vi "Teleop.vi"(10 "Match Info":T1={"Autonomous Elapsed Seconds"=0.0, "TeleOp Elapsed Seconds"=0.0, "Disabled Elapsed Seconds"=0.0, "Visited Autonomous"=FALSE, "Visited TeleOp"=FALSE, "Visited Disabled"=FALSE, "Autonomous Settings"={"Autonomous Style"=enum."Independent", "VI Refnum"=refnum}}, 11 "Call Context":T2) -> ()   [LabVIEW 2018]
doc: "This VI is called for each enabled TeleOp packet received from the DS. It is typically used to read from joysticks and other inputs and update I/O or setpoints for timed control loops. It should complete and return within 20 milliseconds or risk missing DS packets."
uses:
  <vilib>/Rock Robotics/WPI/DriverStation/WPI_DriverStationDerivedRobotMode.ctl
  <vilib>/Rock Robotics/WPI/DriverStation/WPI_DriverStationMatch Info.ctl
  <vilib>/Rock Robotics/WPI/Solenoid/WPI_SolenoidValue.ctl
  Support Code/Climb State Machine Enum.ctl
  Framework/Robot Global Data.vi
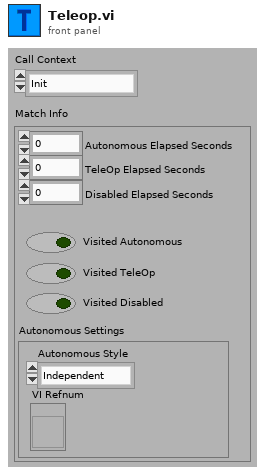
[diagram p1: front panel]
types:
  T1 = typedef "WPI_DriverStationMatch Info.ctl" = cluster{"Autonomous Elapsed Seconds":dbl, "TeleOp Elapsed Seconds":dbl, "Disabled Elapsed Seconds":dbl, "Visited Autonomous":bool, "Visited TeleOp":bool, "Visited Disabled":bool, "Autonomous Settings":cluster{"Autonomous Style":enum16{"Iterative", "Independent"}, "VI Refnum":refnum<vi>}}
  T2 = typedef "WPI_DriverStationDerivedRobotMode.ctl" = enum16{"Init", "Execute", "Stop"}
  T3 = typedef "WPI_SolenoidValue.ctl" = enum16{"Off", "On", "Forward", "Reverse"}
  T4 = typedef "Command Status Info.ctl" = cluster{"Name":string, "Status":T5, "notifier out":T6}
  T5 = typedef "Completion Status.ctl" = enum16{"Successful", "Aborted", "Incomplete"}
  T6 = typedef "Completion Notifier.ctl" = refnum<notifier>
  T7 = typedef "Climb State Machine Enum.ctl" = enum16{"Raise the front of the Robot", "Drive the front forward", "Lift the front pistons", "Lift the back of the Robot", "Drive the back of the robot forward", "Lift the back pistons", "Drive Forward", "Exit"}
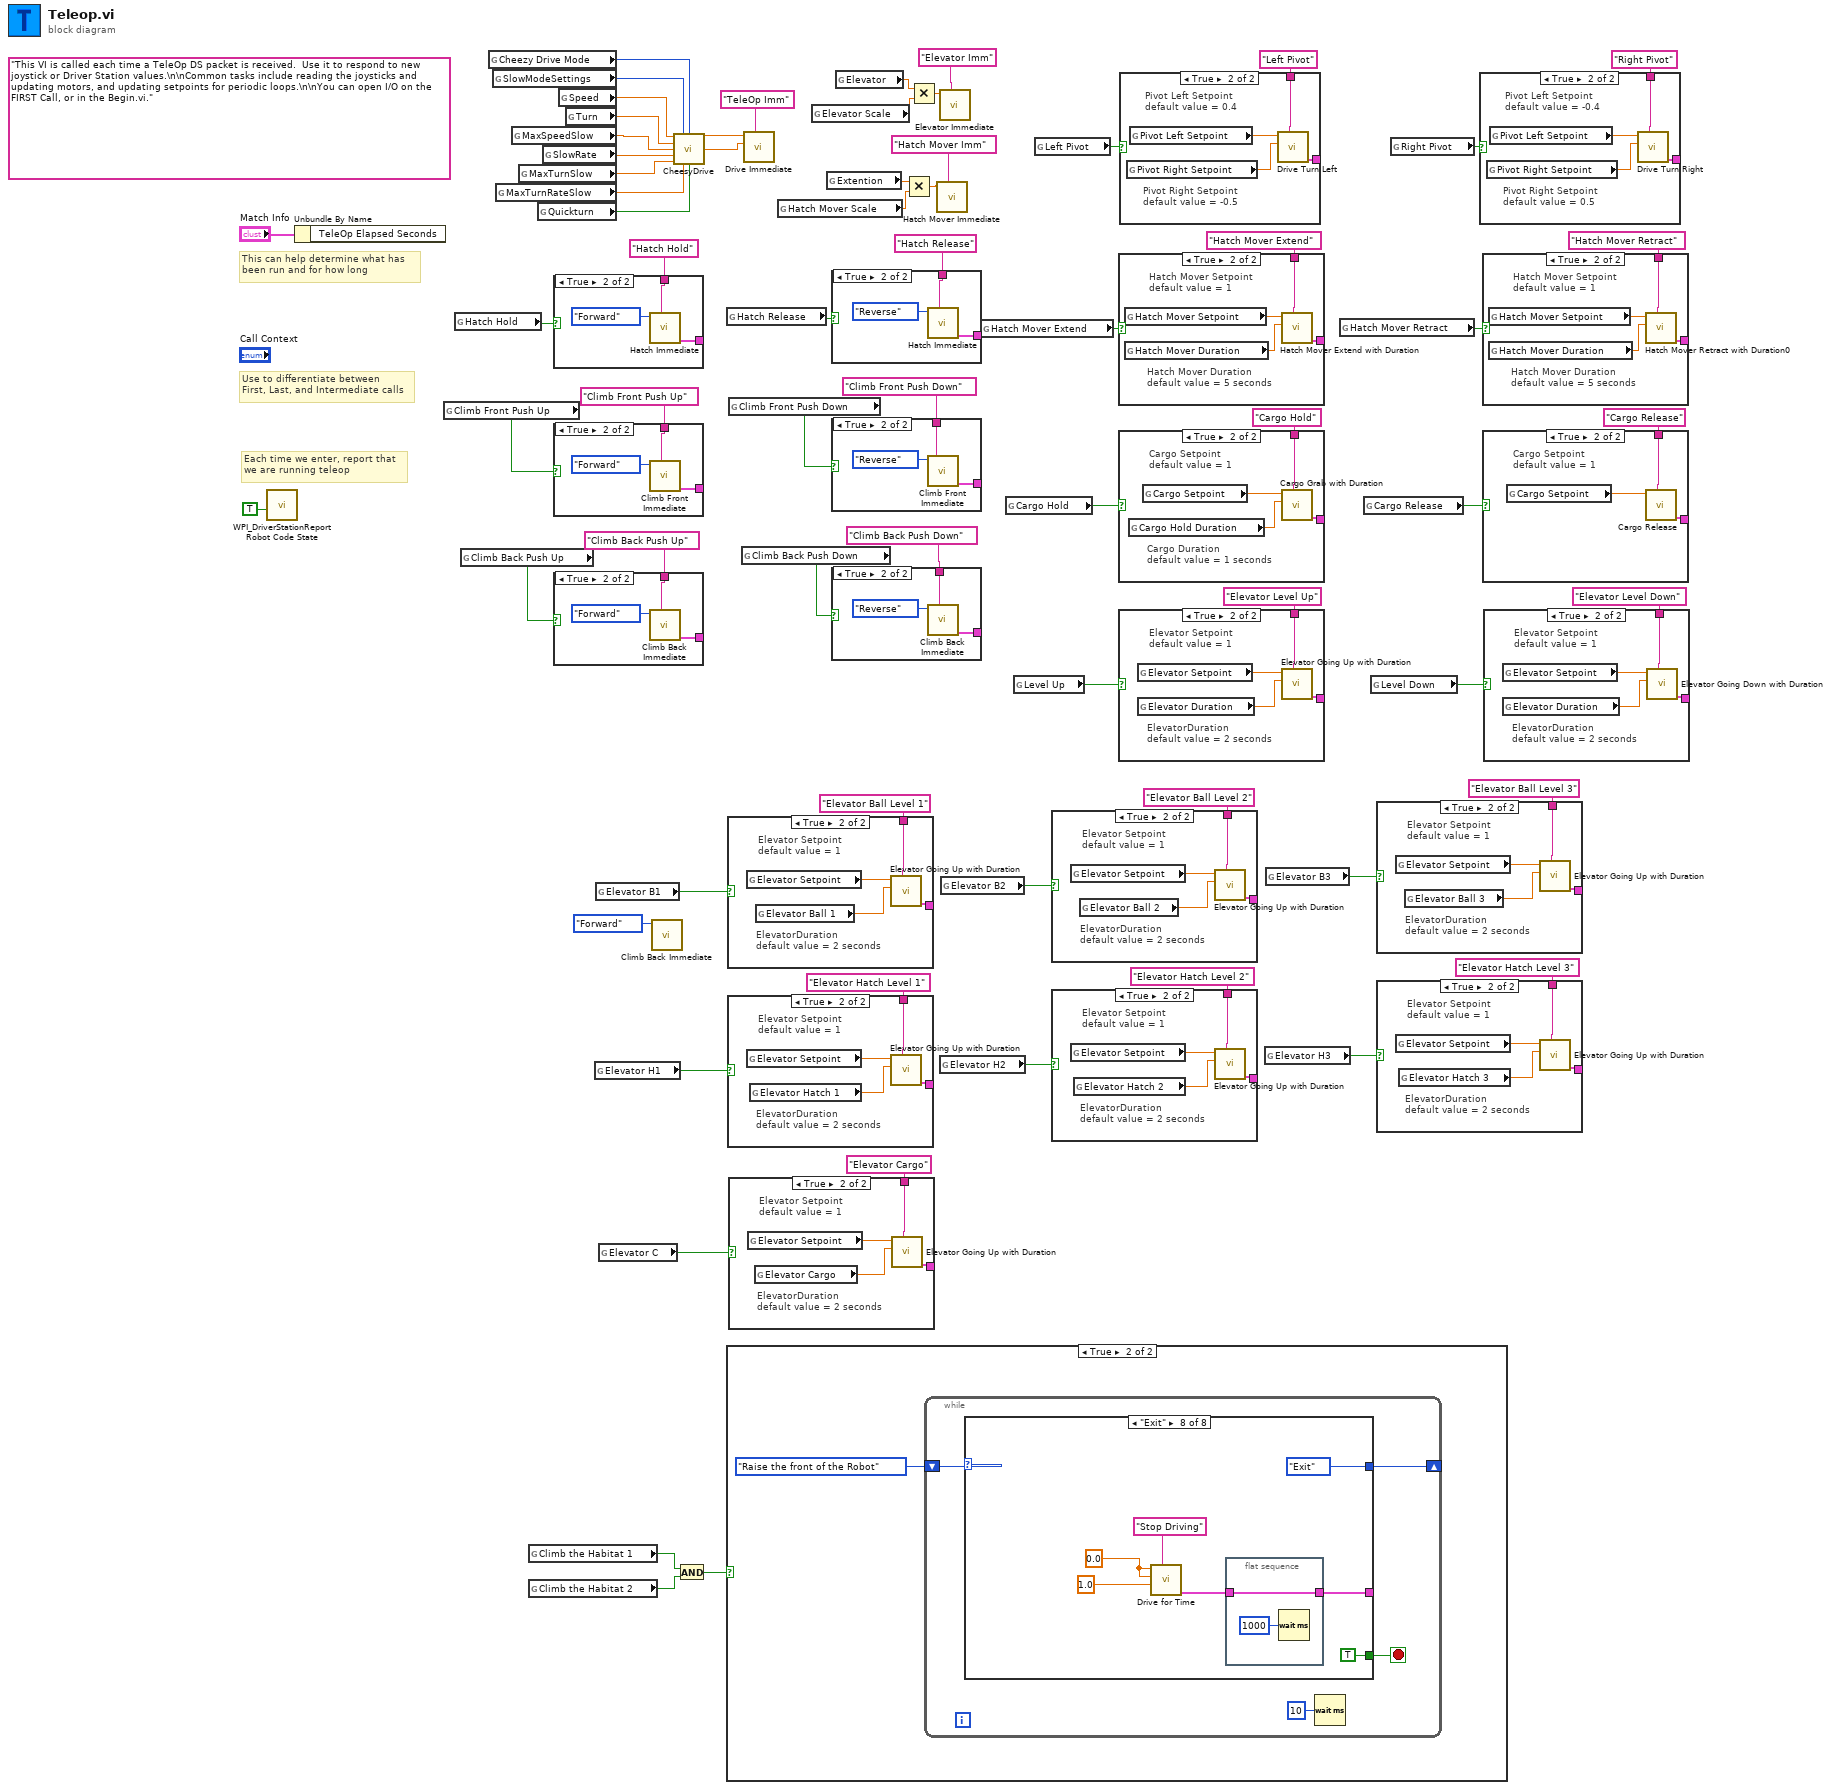
[diagram p0: block diagram]
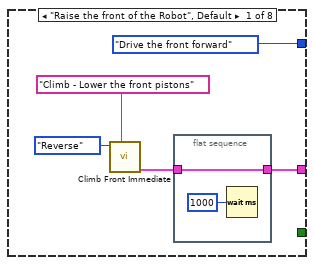
[diagram p3: hidden frame]
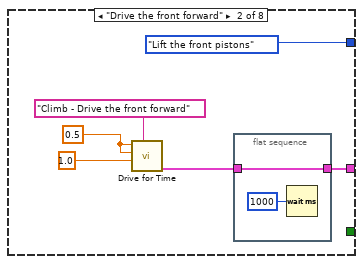
[diagram p4: hidden frame]
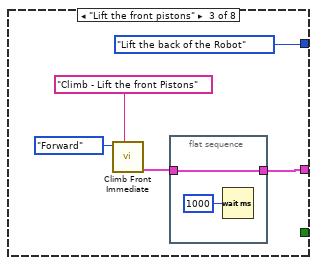
[diagram p5: hidden frame]
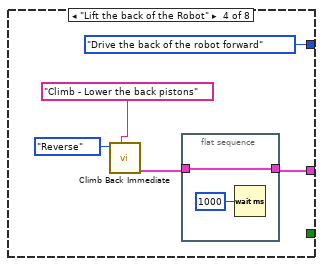
[diagram p6: hidden frame]
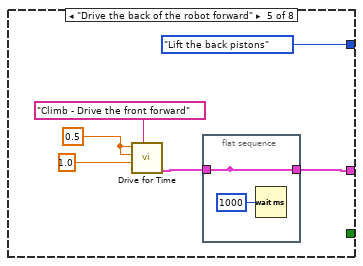
[diagram p7: hidden frame]
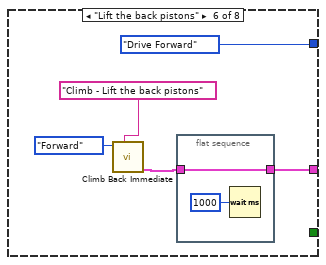
[diagram p8: hidden frame]
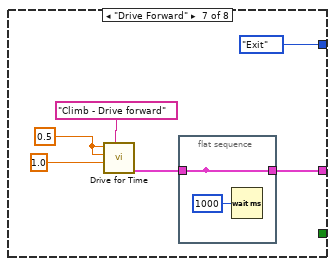
[diagram p9: hidden frame]
diagram:
  (unwired) "This VI is called each time a TeleOp DS packet is received.  Use it to respond to new joystick or Driver Station values.\n\nCommon tasks include reading the joysticks and updating motors, and updating setpoints for periodic loops.\n\nYou can open I/O on the FIRST Call, or in the Begin.vi."
  # "Each time we enter, report that\nwe are running teleop"
  # "Use to differentiate between\nFirst, Last, and Intermediate calls"
  # "This can help determine what has\nbeen run and for how long"
  n1 = call <vilib>:"WPI_DriverStationReport Robot Code State.vi"("TeleOp"=TRUE ("Autonomous")) -> ()  [unwired: 10 in, 1 out]
  n2 = Unbundle By Name("Match Info") -> ()  [unwired: 1 out]
  n3 = global read "Robot Global Data.vi" "Climb Front Push Up"() -> (w60:bool)
  n4 = global read "Robot Global Data.vi" "Hatch Hold"() -> (w64:bool)
  n5 = global read "Robot Global Data.vi" "Climb Back Push Up"() -> (w57:bool)
  n6 = global read "Robot Global Data.vi" "Cheezy Drive Mode"() -> (w37:u32)
  n7 = global read "Robot Global Data.vi" "SlowModeSettings"() -> (w36:i32)
  n8 = global read "Robot Global Data.vi" "MaxTurnRateSlow"() -> (w30:dbl)
  n9 = global read "Robot Global Data.vi" "MaxSpeedSlow"() -> (w33:dbl)
  n10 = global read "Robot Global Data.vi" "MaxTurnSlow"() -> (w31:dbl)
  n11 = global read "Robot Global Data.vi" "Climb the Habitat 1"() -> (w2:bool)
  n12 = global read "Robot Global Data.vi" "Climb the Habitat 2"() -> (w1:bool)
  n13 = global read "Robot Global Data.vi" "Quickturn"() -> (w29:bool)
  n14 = global read "Robot Global Data.vi" "SlowRate"() -> (w32:dbl)
  n15 = case shown="True" w64 {
    tunnel: [_ w70] -> _
    tunnel: "Hatch Hold" ("Description") -> [_ w69]
    frame False {
    }
    frame True {
      n16 = call "Hatch Immediate.vi"("Description"=w69, "Action"=WPI_SolenoidValue."Forward") -> ("Command Info Out"=w70:T4)  [unwired: 9 in]
    }
  }
  n17 = case shown="True" w60 {
    tunnel: [_ w73] -> _
    tunnel: "Climb Front Push Up" ("Description") -> [_ w72]
    frame False {
    }
    frame True {
      n18 = call "Climb Front Immediate.vi"("Description"=w72, "Action"=WPI_SolenoidValue."Forward") -> ("Command Info Out"=w73:T4)  [unwired: 9 in]
    }
  }
  n19 = case shown="True" w57 {
    tunnel: [_ w77] -> _
    tunnel: "Climb Back Push Up" ("Description") -> [_ w76]
    frame False {
    }
    frame True {
      n20 = call "Climb Back Immediate.vi"("Description"=w76, "Relay Value"=WPI_SolenoidValue."Forward" ("Action")) -> ("Command Info Out"=w77:T4)  [unwired: 9 in]
    }
  }
  n21 = global read "Robot Global Data.vi" "Speed"() -> (w35:dbl)
  n22 = global read "Robot Global Data.vi" "Turn"() -> (w34:dbl)
  n23 = global read "Robot Global Data.vi" "Elevator H1"() -> (w8:bool)
  n24 = global read "Robot Global Data.vi" "Elevator B1"() -> (w17:bool)
  n25 = global read "Robot Global Data.vi" "Elevator C"() -> (w5:bool)
  n26 = call "Climb Back Immediate.vi"("Relay Value"=WPI_SolenoidValue."Forward" ("Action")) -> ()  [unwired: 10 in, 1 out]
  n27 = call "CheesyDrive.vi"("Throttle"=w35, "SlowModeSettings"=w36, "SlowMode"=w37, "Wheel"=w34, "MaxSpeedSlow"=w33, "SlowRate"=w32, "MaxTurnSlow"=w31, "MaxTurnRateSlow"=w30, "Quickturn"=w29) -> ("Left PWM"=w28:dbl, "Right PWM"=w27:dbl)  [unwired: 5 in]
  n28 = And(x=w2, y=w1) -> (x .and. y?=w3:bool)
  n29 = global read "Robot Global Data.vi" "Hatch Release"() -> (w63:bool)
  n30 = case shown="True" w3 {
    frame False {
    }
    frame True {
      n31 = while {
        shift-right: [w80] -> _
        shift-left: Climb_State_Machine_Enum."Raise the front of the Robot" -> [w82]
        stop <- w79 stop-if-true
        n32 = case shown="\"Exit\"" w82 {
          tunnel: [w83 w90 w98 w105 w112 w120 w128 w137] -> _
          tunnel: [Climb_State_Machine_Enum."Drive the front forward" Climb_State_Machine_Enum."Lift the front pistons" Climb_State_Machine_Enum."Lift the back of the Robot" Climb_State_Machine_Enum."Drive the back of the robot forward" Climb_State_Machine_Enum."Lift the back pistons" Climb_State_Machine_Enum."Drive Forward" Climb_State_Machine_Enum."Exit" Climb_State_Machine_Enum."Exit"] -> w80
          tunnel: [_ _ _ _ _ _ _ TRUE] -> w79
          frame "Raise the front of the Robot", Default {
            n33 = call "Climb Front Immediate.vi"("Description"="Climb - Lower the front pistons", "Action"=WPI_SolenoidValue."Reverse") -> ("Command Info Out"=w84:T4)  [unwired: 9 in]
            n34 = flat-sequence {
              tunnel: [w89] -> w83
              tunnel: w84 -> [w89]
              frame #0 {
                n35 = Wait (ms)(milliseconds to wait=u32 1000) -> ()  [unwired: 1 out]
              }
            }
          }
          frame "Drive the front forward" {
            w95 = 0.5 ("Left Speed")
            n36 = call "Drive for Time.vi"("Description"="Climb - Drive the front forward", "Seconds"=1.0, "Right Speed"=w95, "Left Speed"=w95) -> ("Command Info Out"=w91:T4)  [unwired: 7 in]
            n37 = flat-sequence {
              tunnel: [w97] -> w90
              tunnel: w91 -> [w97]
              frame #0 {
                n38 = Wait (ms)(milliseconds to wait=u32 1000) -> ()  [unwired: 1 out]
              }
            }
          }
          frame "Lift the front pistons" {
            n39 = call "Climb Front Immediate.vi"("Description"="Climb - Lift the front Pistons", "Action"=WPI_SolenoidValue."Forward") -> ("Command Info Out"=w99:T4)  [unwired: 9 in]
            n40 = flat-sequence {
              tunnel: [w104] -> w98
              tunnel: w99 -> [w104]
              frame #0 {
                n41 = Wait (ms)(milliseconds to wait=u32 1000) -> ()  [unwired: 1 out]
              }
            }
          }
          frame "Lift the back of the Robot" {
            n42 = call "Climb Back Immediate.vi"("Description"="Climb - Lower the back pistons", "Relay Value"=WPI_SolenoidValue."Reverse" ("Action")) -> ("Command Info Out"=w106:T4)  [unwired: 9 in]
            n43 = flat-sequence {
              tunnel: [w111] -> w105
              tunnel: w106 -> [w111]
              frame #0 {
                n44 = Wait (ms)(milliseconds to wait=u32 1000) -> ()  [unwired: 1 out]
              }
            }
          }
          frame "Drive the back of the robot forward" {
            w117 = 0.5 ("Left Speed")
            n45 = call "Drive for Time.vi"("Description"="Climb - Drive the front forward", "Seconds"=1.0, "Right Speed"=w117, "Left Speed"=w117) -> ("Command Info Out"=w113:T4)  [unwired: 7 in]
            n46 = flat-sequence {
              tunnel: [w118] -> _
              tunnel: w113 -> [w118]
              tunnel: [w118] -> w112
              frame #0 {
                n47 = Wait (ms)(milliseconds to wait=u32 1000) -> ()  [unwired: 1 out]
              }
            }
          }
          frame "Lift the back pistons" {
            n48 = call "Climb Back Immediate.vi"("Description"="Climb - Lift the back pistons", "Relay Value"=WPI_SolenoidValue."Forward" ("Action")) -> ("Command Info Out"=w121:T4)  [unwired: 9 in]
            n49 = flat-sequence {
              tunnel: [w126] -> w120
              tunnel: w121 -> [w126]
              frame #0 {
                n50 = Wait (ms)(milliseconds to wait=u32 1000) -> ()  [unwired: 1 out]
              }
            }
          }
          frame "Drive Forward" {
            w132 = 0.5 ("Left Speed")
            n51 = call "Drive for Time.vi"("Description"="Climb - Drive forward", "Seconds"=1.0, "Right Speed"=w132, "Left Speed"=w132) -> ("Command Info Out"=w129:T4)  [unwired: 7 in]
            n52 = flat-sequence {
              tunnel: [w133] -> _
              tunnel: w129 -> [w133]
              tunnel: [w133] -> w128
              frame #0 {
                n53 = Wait (ms)(milliseconds to wait=u32 1000) -> ()  [unwired: 1 out]
              }
            }
          }
          frame "Exit" {
            w141 = 0.0 ("Left Speed")
            n54 = call "Drive for Time.vi"("Description"="Stop Driving", "Seconds"=1.0, "Right Speed"=w141, "Left Speed"=w141) -> ("Command Info Out"=w138:T4)  [unwired: 7 in]
            n55 = flat-sequence {
              tunnel: w138 -> [w142]
              tunnel: [w142] -> w137
              frame #0 {
                n56 = Wait (ms)(milliseconds to wait=u32 1000) -> ()  [unwired: 1 out]
              }
            }
          }
        }
        n57 = Wait (ms)(milliseconds to wait=u32 10) -> ()  [unwired: 1 out]
      }
    }
  }
  n58 = case shown="True" w17 {
    tunnel: "Elevator Ball Level 1" ("Description") -> [_ w147]
    tunnel: [_ w144] -> _
    frame False {
    }
    frame True {
      # "ElevatorDuration\ndefault value = 2 seconds"
      # "Elevator Setpoint\ndefault value = 1"
      n59 = global read "Robot Global Data.vi" "Elevator Setpoint"() -> (w146:dbl)
      n60 = global read "Robot Global Data.vi" "Elevator Ball 1"() -> (w145:dbl)
      n61 = call "Elevator Going Up with Duration.vi"("Description"=w147, "Duration (s)"=w145, "Setpoint"=w146) -> ("Command Info Out"=w144:T4)  [unwired: 8 in]
    }
  }
  n62 = case shown="True" w8 {
    tunnel: "Elevator Hatch Level 1" ("Description") -> [_ w151]
    tunnel: [_ w148] -> _
    frame False {
    }
    frame True {
      # "ElevatorDuration\ndefault value = 2 seconds"
      # "Elevator Setpoint\ndefault value = 1"
      n63 = global read "Robot Global Data.vi" "Elevator Setpoint"() -> (w150:dbl)
      n64 = global read "Robot Global Data.vi" "Elevator Hatch 1"() -> (w149:dbl)
      n65 = call "Elevator Going Up with Duration.vi"("Description"=w151, "Duration (s)"=w149, "Setpoint"=w150) -> ("Command Info Out"=w148:T4)  [unwired: 8 in]
    }
  }
  n66 = global read "Robot Global Data.vi" "Climb Front Push Down"() -> (w61:bool)
  n67 = case shown="True" w5 {
    tunnel: "Elevator Cargo" ("Description") -> [_ w155]
    tunnel: [_ w152] -> _
    frame False {
    }
    frame True {
      # "ElevatorDuration\ndefault value = 2 seconds"
      # "Elevator Setpoint\ndefault value = 1"
      n68 = global read "Robot Global Data.vi" "Elevator Setpoint"() -> (w154:dbl)
      n69 = global read "Robot Global Data.vi" "Elevator Cargo"() -> (w153:dbl)
      n70 = call "Elevator Going Up with Duration.vi"("Description"=w155, "Duration (s)"=w153, "Setpoint"=w154) -> ("Command Info Out"=w152:T4)  [unwired: 8 in]
    }
  }
  n71 = global read "Robot Global Data.vi" "Climb Back Push Down"() -> (w56:bool)
  n72 = call "Drive Immediate.vi"("Description"="TeleOp Imm", "Right Setpoint"=w27, "Left Setpoint"=w28) -> ()  [unwired: 8 in, 1 out]
  n73 = global read "Robot Global Data.vi" "Hatch Mover Scale"() -> (w22:dbl)
  n74 = global read "Robot Global Data.vi" "Elevator Scale"() -> (w19:dbl)
  n75 = global read "Robot Global Data.vi" "Extention"() -> (w23:dbl)
  n76 = case shown="True" w63 {
    tunnel: [_ w157] -> _
    tunnel: "Hatch Release" ("Description") -> [_ w156]
    frame False {
    }
    frame True {
      n77 = call "Hatch Immediate.vi"("Description"=w156, "Action"=WPI_SolenoidValue."Reverse") -> ("Command Info Out"=w157:T4)  [unwired: 9 in]
    }
  }
  n78 = case shown="True" w61 {
    tunnel: [_ w160] -> _
    tunnel: "Climb Front Push Down" ("Description") -> [_ w159]
    frame False {
    }
    frame True {
      n79 = call "Climb Front Immediate.vi"("Description"=w159, "Action"=WPI_SolenoidValue."Reverse") -> ("Command Info Out"=w160:T4)  [unwired: 9 in]
    }
  }
  n80 = case shown="True" w56 {
    tunnel: [_ w164] -> _
    tunnel: "Climb Back Push Down" ("Description") -> [_ w163]
    frame False {
    }
    frame True {
      n81 = call "Climb Back Immediate.vi"("Description"=w163, "Relay Value"=WPI_SolenoidValue."Reverse" ("Action")) -> ("Command Info Out"=w164:T4)  [unwired: 9 in]
    }
  }
  n82 = global read "Robot Global Data.vi" "Elevator"() -> (w20:dbl)
  n83 = Multiply(x=w23, y=w22) -> (x*y=w24:dbl)
  n84 = Multiply(x=w20, y=w19) -> (x*y=w21:dbl)
  n85 = call "Hatch Mover Immediate.vi"("Description"="Hatch Mover Imm", "Setpoint"=w24) -> ()  [unwired: 9 in, 1 out]
  n86 = call "Elevator Immediate.vi"("Description"="Elevator Imm", "Setpoint"=w21) -> ()  [unwired: 9 in, 1 out]
  n87 = global read "Robot Global Data.vi" "Elevator H2"() -> (w9:bool)
  n88 = global read "Robot Global Data.vi" "Elevator B2"() -> (w16:bool)
  n89 = global read "Robot Global Data.vi" "Hatch Mover Extend"() -> (w49:bool)
  n90 = global read "Robot Global Data.vi" "Cargo Hold"() -> (w44:bool)
  n91 = global read "Robot Global Data.vi" "Level Up"() -> (w41:bool)
  n92 = global read "Robot Global Data.vi" "Left Pivot"() -> (w52:bool)
  n93 = case shown="True" w16 {
    tunnel: "Elevator Ball Level 2" ("Description") -> [_ w168]
    tunnel: [_ w165] -> _
    frame False {
    }
    frame True {
      # "ElevatorDuration\ndefault value = 2 seconds"
      # "Elevator Setpoint\ndefault value = 1"
      n94 = global read "Robot Global Data.vi" "Elevator Setpoint"() -> (w167:dbl)
      n95 = global read "Robot Global Data.vi" "Elevator Ball 2"() -> (w166:dbl)
      n96 = call "Elevator Going Up with Duration.vi"("Description"=w168, "Duration (s)"=w166, "Setpoint"=w167) -> ("Command Info Out"=w165:T4)  [unwired: 8 in]
    }
  }
  n97 = case shown="True" w9 {
    tunnel: "Elevator Hatch Level 2" ("Description") -> [_ w172]
    tunnel: [_ w169] -> _
    frame False {
    }
    frame True {
      # "ElevatorDuration\ndefault value = 2 seconds"
      # "Elevator Setpoint\ndefault value = 1"
      n98 = global read "Robot Global Data.vi" "Elevator Setpoint"() -> (w171:dbl)
      n99 = global read "Robot Global Data.vi" "Elevator Hatch 2"() -> (w170:dbl)
      n100 = call "Elevator Going Up with Duration.vi"("Description"=w172, "Duration (s)"=w170, "Setpoint"=w171) -> ("Command Info Out"=w169:T4)  [unwired: 8 in]
    }
  }
  n101 = case shown="True" w49 {
    tunnel: "Hatch Mover Extend" ("Description") -> [_ w176]
    tunnel: [_ w173] -> _
    frame False {
    }
    frame True {
      # "Hatch Mover Duration\ndefault value = 5 seconds"
      # "Hatch Mover Setpoint\ndefault value = 1"
      n102 = global read "Robot Global Data.vi" "Hatch Mover Setpoint"() -> (w175:dbl)
      n103 = global read "Robot Global Data.vi" "Hatch Mover Duration"() -> (w174:dbl)
      n104 = call "Hatch Mover Extend with Duration.vi"("Description"=w176, "Duration (s)"=w174, "Setpoint"=w175) -> ("Command Info Out"=w173:T4)  [unwired: 8 in]
    }
  }
  n105 = case shown="True" w44 {
    tunnel: "Cargo Hold" ("Description") -> [_ w180]
    tunnel: [_ w177] -> _
    frame False {
    }
    frame True {
      # "Cargo Duration\ndefault value = 1 seconds"
      # "Cargo Setpoint\ndefault value = 1"
      n106 = global read "Robot Global Data.vi" "Cargo Hold Duration"() -> (w178:dbl)
      n107 = global read "Robot Global Data.vi" "Cargo Setpoint"() -> (w179:dbl)
      n108 = call "Cargo Grab with Duration.vi"("Description"=w180, "Duration (s)"=w178, "Setpoint"=w179) -> ("Command Info Out"=w177:T4)  [unwired: 8 in]
    }
  }
  n109 = case shown="True" w41 {
    tunnel: "Elevator Level Up" ("Description") -> [_ w184]
    tunnel: [_ w181] -> _
    frame False {
    }
    frame True {
      # "ElevatorDuration\ndefault value = 2 seconds"
      # "Elevator Setpoint\ndefault value = 1"
      n110 = global read "Robot Global Data.vi" "Elevator Setpoint"() -> (w183:dbl)
      n111 = global read "Robot Global Data.vi" "Elevator Duration"() -> (w182:dbl)
      n112 = call "Elevator Going Up with Duration.vi"("Description"=w184, "Duration (s)"=w182, "Setpoint"=w183) -> ("Command Info Out"=w181:T4)  [unwired: 8 in]
    }
  }
  n113 = case shown="True" w52 {
    tunnel: "Left Pivot" ("Description") -> [_ w188]
    tunnel: [_ w185] -> _
    frame False {
    }
    frame True {
      # "Pivot Right Setpoint\ndefault value = -0.5"
      # "Pivot Left Setpoint\ndefault value = 0.4"
      n114 = global read "Robot Global Data.vi" "Pivot Right Setpoint"() -> (w186:dbl)
      n115 = global read "Robot Global Data.vi" "Pivot Left Setpoint"() -> (w187:dbl)
      n116 = call "Drive Turn Left.vi"("Description"=w188, "Right Setpoint"=w186, "Left Setpoint"=w187) -> ("Command Info Out"=w185:T4)  [unwired: 8 in]
    }
  }
  n117 = global read "Robot Global Data.vi" "Elevator H3"() -> (w12:bool)
  n118 = global read "Robot Global Data.vi" "Elevator B3"() -> (w13:bool)
  n119 = global read "Robot Global Data.vi" "Hatch Mover Retract"() -> (w46:bool)
  n120 = global read "Robot Global Data.vi" "Cargo Release"() -> (w43:bool)
  n121 = global read "Robot Global Data.vi" "Level Down"() -> (w38:bool)
  n122 = case shown="True" w13 {
    tunnel: "Elevator Ball Level 3" ("Description") -> [_ w192]
    tunnel: [_ w189] -> _
    frame False {
    }
    frame True {
      # "ElevatorDuration\ndefault value = 2 seconds"
      # "Elevator Setpoint\ndefault value = 1"
      n123 = global read "Robot Global Data.vi" "Elevator Setpoint"() -> (w191:dbl)
      n124 = global read "Robot Global Data.vi" "Elevator Ball 3"() -> (w190:dbl)
      n125 = call "Elevator Going Up with Duration.vi"("Description"=w192, "Duration (s)"=w190, "Setpoint"=w191) -> ("Command Info Out"=w189:T4)  [unwired: 8 in]
    }
  }
  n126 = case shown="True" w12 {
    tunnel: "Elevator Hatch Level 3" ("Description") -> [_ w196]
    tunnel: [_ w193] -> _
    frame False {
    }
    frame True {
      # "ElevatorDuration\ndefault value = 2 seconds"
      # "Elevator Setpoint\ndefault value = 1"
      n127 = global read "Robot Global Data.vi" "Elevator Setpoint"() -> (w195:dbl)
      n128 = global read "Robot Global Data.vi" "Elevator Hatch 3"() -> (w194:dbl)
      n129 = call "Elevator Going Up with Duration.vi"("Description"=w196, "Duration (s)"=w194, "Setpoint"=w195) -> ("Command Info Out"=w193:T4)  [unwired: 8 in]
    }
  }
  n130 = global read "Robot Global Data.vi" "Right Pivot"() -> (w51:bool)
  n131 = case shown="True" w51 {
    tunnel: "Right Pivot" ("Description") -> [_ w200]
    tunnel: [_ w197] -> _
    frame False {
    }
    frame True {
      # "Pivot Right Setpoint\ndefault value = 0.5"
      # "Pivot Left Setpoint\ndefault value = -0.4"
      n132 = global read "Robot Global Data.vi" "Pivot Right Setpoint"() -> (w198:dbl)
      n133 = global read "Robot Global Data.vi" "Pivot Left Setpoint"() -> (w199:dbl)
      n134 = call "Drive Turn Right.vi"("Description"=w200, "Right Setpoint"=w198, "Left Setpoint"=w199) -> ("Command Info Out"=w197:T4)  [unwired: 8 in]
    }
  }
  n135 = case shown="True" w46 {
    tunnel: "Hatch Mover Retract" ("Description") -> [_ w204]
    tunnel: [_ w201] -> _
    frame False {
    }
    frame True {
      # "Hatch Mover Duration\ndefault value = 5 seconds"
      # "Hatch Mover Setpoint\ndefault value = 1"
      n136 = global read "Robot Global Data.vi" "Hatch Mover Setpoint"() -> (w203:dbl)
      n137 = global read "Robot Global Data.vi" "Hatch Mover Duration"() -> (w202:dbl)
      n138 = call "Hatch Mover Retract with Duration0.vi"("Description"=w204, "Duration (s)"=w202, "Setpoint"=w203) -> ("Command Info Out"=w201:T4)  [unwired: 8 in]
    }
  }
  n139 = case shown="True" w43 {
    tunnel: "Cargo Release" ("Description") -> [_ w207]
    tunnel: [_ w205] -> _
    frame False {
    }
    frame True {
      # "Cargo Setpoint\ndefault value = 1"
      n140 = global read "Robot Global Data.vi" "Cargo Setpoint"() -> (w206:dbl)
      n141 = call "Cargo Release.vi"("Description"=w207, "Setpoint"=w206) -> ("Command Info Out"=w205:T4)  [unwired: 9 in]
    }
  }
  n142 = case shown="True" w38 {
    tunnel: "Elevator Level Down" ("Description") -> [_ w211]
    tunnel: [_ w208] -> _
    frame False {
    }
    frame True {
      # "ElevatorDuration\ndefault value = 2 seconds"
      # "Elevator Setpoint\ndefault value = 1"
      n143 = global read "Robot Global Data.vi" "Elevator Setpoint"() -> (w210:dbl)
      n144 = global read "Robot Global Data.vi" "Elevator Duration"() -> (w209:dbl)
      n145 = call "Elevator Going Down with Duration.vi"("Description"=w211, "Duration (s)"=w209, "Setpoint"=w210) -> ("Command Info Out"=w208:T4)  [unwired: 8 in]
    }
  }
